vi "Begin.vi"   [LabVIEW 2012]
doc: "Called before other user functions, this VI is expected to open initial I/O refnums, load in file data, and do all program initialization. Notice that the <B>error out</B> terminal is simply used for data flow. Wiring it to other structures or subVIs ensures that this VI runs first."
uses:
  <vilib>/Rock Robotics/SystemInterfaces/Typedef/FPGA_TypedefAnalogModule.ctl
  <vilib>/Rock Robotics/SystemInterfaces/AI/FPGA_AIChannel.ctl
  <vilib>/Rock Robotics/SystemInterfaces/DIO/FPGA_DIOPWMChannel.ctl
  <vilib>/Rock Robotics/SystemInterfaces/Typedef/FPGA_TypedefDigitalModule.ctl
  <vilib>/Rock Robotics/SystemInterfaces/DIO/FPGA_DIOChannel.ctl
  <vilib>/Rock Robotics/WPI/Joystick/WPI_JoystickDeviceEnum.ctl
  <vilib>/Rock Robotics/SystemInterfaces/DIO/FPGA_DIORelayChannel.ctl
  <vilib>/Rock Robotics/WPI/Relay/WPI_RelayDirection.ctl
  <vilib>/Rock Robotics/WPI/SafetyOutput/WPI_SafetyOutputConfigMenu.ctl
  <vilib>/Rock Robotics/WPI/MotorControl/WPI_MotorControlOpen Jaguar.vi
  <vilib>/Rock Robotics/WPI/MotorControl/WPI_MotorControlOpen Victor.vi
  <vilib>/Rock Robotics/WPI/RobotDrive/WPI_RobotDriveOpen2MotorWithJaguar.vi
types:
  T1 = typedef "WPI_SafetyOutputConfigMenu.ctl" = enum16{"Enable", "Disable"}
  T2 = typedef "FPGA_DIOPWMChannel.ctl" = enum8{"PWM 1", "PWM 2", "PWM 3", "PWM 4", "PWM 5", "PWM 6", "PWM 7", "PWM 8", "PWM 9", "PWM 10", "Invalid"}
  T3 = typedef "WPI_RobotDriveDevRef.ctl" = cluster{"DevStatus":errorcluster, "Motors[]":T4[], "Square Inputs":bool, "Max Output":dbl, "Isochronous":bool}
  T4 = typedef "WPI_MotorControlDeviceRef.ctl" = cluster{"DeviceStatus":errorcluster, "Type":enum16{"PWM", "CAN"}, "PWM":cluster{"Digital Module":T5, "PWM Channel":T2, "DeadBand":T6}, "CAN":cluster{"Device Number":u8, "Control Mode":T7, "Semaphore":T8, "Max Vout":dbl}, "Invert":bool, "TransformRef":T9, "InvTransformRef":T9}
  T5 = typedef "FPGA_TypedefDigitalModule.ctl" = enum16{"Digital Module 1", "Digital Module 2"}
  T6 = typedef "WPI_PWMDeadband.ctl" = cluster{"Name":string, "maxPositivePwm":i32, "minPositivePwm":i32, "centerPwm":i32, "maxNegativePwm":i32, "minNegativePwm":i32, "angularRange":u16}
  T7 = typedef "WPI_CANJaguar_ControlMode.ctl" = enum8{"Percent VBus", "Current", "Speed", "Position", "Voltage"}
  T8 = typedef "Semaphore RefNum" = refnum<k1>
  T9 = typedef "WPI_PWMTransform_ConPane.ctl" = refnum<vi>
  T10 = typedef "WPI_RelayDirection.ctl" = enum16{"Both directions", "Forward only", "Reverse only"}
  T11 = typedef "FPGA_DIORelayChannel.ctl" = enum8{"Relay 1", "Relay 2", "Relay 3", "Relay 4", "Relay 5", "Relay 6", "Relay 7", "Relay 8", "Invalid"}
  T12 = typedef "WPI_ServoDeviceRef.ctl" = cluster{"DeviceStatus":errorcluster, "Digital Module":T5, "PWM Channel":T2, "DeadBand":T6}
  T13 = typedef "WPI_RelayDevRef.ctl" = cluster{"DevStatus":errorcluster, "Relay Channel":T11, "Digital Module":T5, "Relay Direction":T10}
  T14 = typedef "WPI_JoystickDeviceEnum.ctl" = enum16{"USB 1", "USB 2", "USB 3", "USB 4", "Kinect 1", "Kinect 2"}
  T15 = typedef "WPI_JoystickDevRef.ctl" = cluster{"Device":T14}
  T16 = typedef "FPGA_DIOChannel.ctl" = enum8{"DIO 1", "DIO 2", "DIO 3", "DIO 4", "DIO 5", "DIO 6", "DIO 7", "DIO 8", "DIO 9", "DIO 10", "DIO 11", "DIO 12", "DIO 13", "DIO 14", "Invalid"}
  T17 = typedef "WPI_DigitalInputDevRef.ctl" = cluster{"DevStatus":errorcluster, "DIO Channel":T16, "Digital Module":T5}
  T18 = typedef "FPGA_AIChannel.ctl" = enum8{"AI 1", "AI 2", "AI 3", "AI 4", "AI 5", "AI 6", "AI 7", "AI 8", "Invalid"}
  T19 = typedef "FPGA_TypedefAnalogModule.ctl" = enum16{"Analog Module 1", "Analog Module 2"}
  T20 = typedef "WPI_AnalogChannelDevRef.ctl" = cluster{"DevStatus":errorcluster, "Analog Module":T19, "Analog Channel":T18}
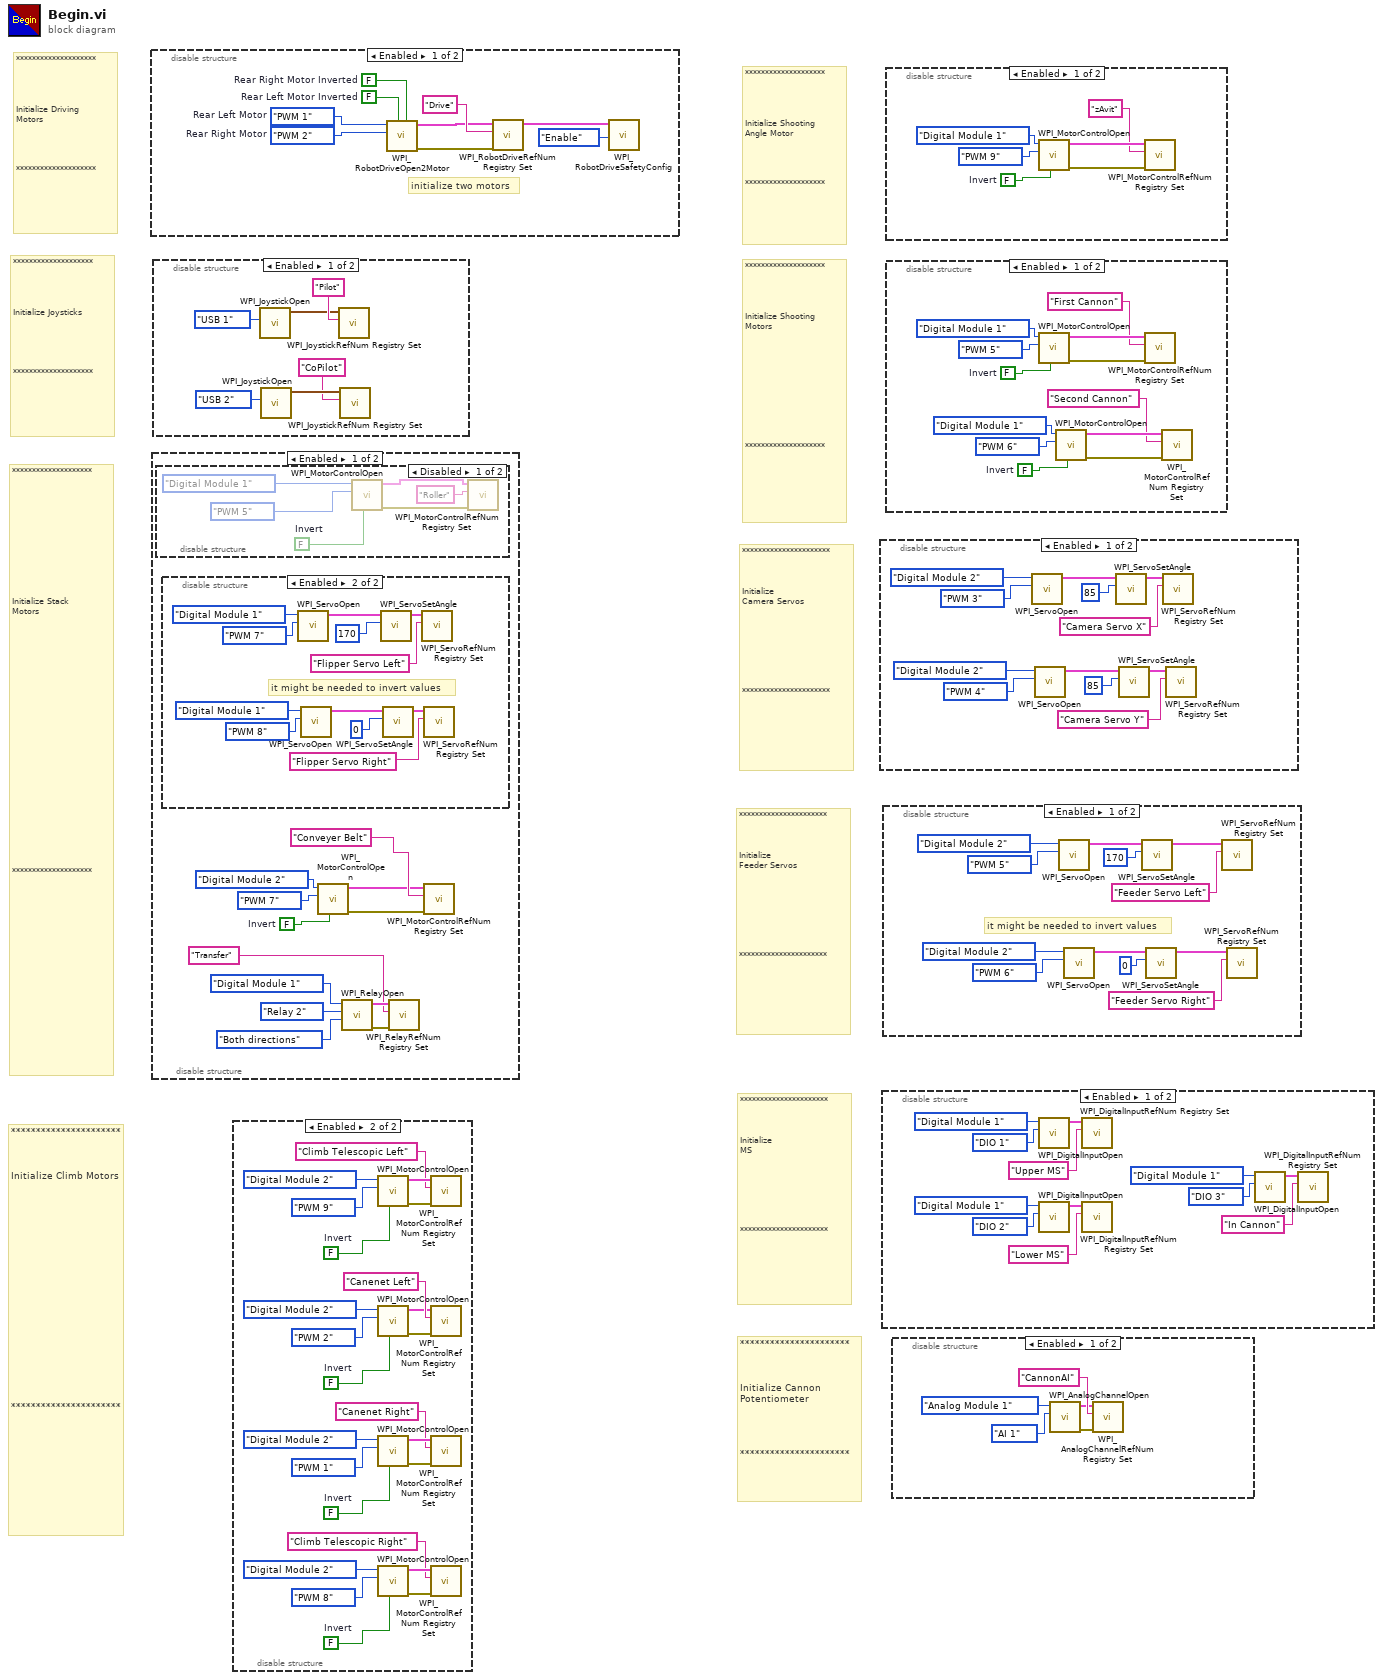
[diagram p0: block diagram]
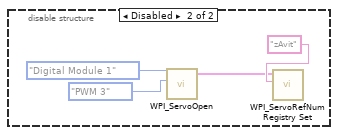
[diagram p7: hidden frame]
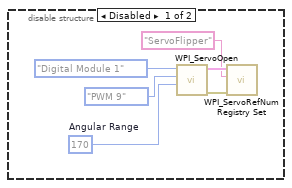
[diagram p11: hidden frame]
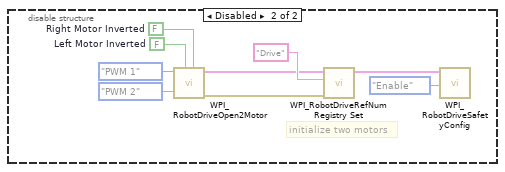
[diagram p13: hidden frame]
diagram:
  # "**********************\n\n\n           \nInitialize Cannon Potentiometer\n\n\n\n\n**********************"
  # "**********************\n\n\n\nInitialize\nMS\n\n\n\n\n\n\n\n**********************"
  # "**********************\n\n\n\nInitialize\nFeeder Servos\n\n\n\n\n\n\n\n\n**********************"
  # "**********************\n\n\n\nInitialize\nCamera Servos\n\n\n\n\n\n\n\n\n**********************"
  # "**********************\n\n\n\nInitialize Climb Motors          \n\n\n\n\n\n\n\n\n\n\n\n\n\n\n\n\n\n\n\n\n**********************"
  # "********************\n\n\n\n\nInitialize Shooting\nAngle Motor\n\n\n\n\n********************"
  # "********************\n\n\n\n\nInitialize Shooting\nMotors\n\n\n\n\n\n\n\n\n\n\n\n********************"
  # "********************\n\n\n\n\n\n\n\n\n\n\n\n\nInitialize Stack \nMotors\n\n\n\n\n\n\n\n\n\n\n\n\n\n\n\n\n\n\n\n\n\n\n\n\n\n********************"
  # "********************\n\n\n\n\nInitialize Driving\nMotors\n\n\n\n\n********************"
  # "********************\n\n\n\n\nInitialize Joysticks\n\n\n\n\n\n********************"
  n1 = disable-structure shown="Enabled" {
    frame Enabled {
      w1 = FPGA_DIOPWMChannel."PWM 2"  # Rear Right Motor
      w2 = FPGA_DIOPWMChannel."PWM 1"  # Rear Left Motor
      w3 = FALSE  # Rear Right Motor Inverted
      w4 = FALSE  # Rear Left Motor Inverted
      # "initialize two motors"
      n2 = call-poly <vilib>:"WPI_RobotDriveOpen2Motor.vi"("Right Motor Inverted"=w3, "Left Motor Inverted"=w4, "Right Motor"=w1, "Left Motor"=w2) -> ("error out"=w5:errorcluster, "RobotDriveDevRef"=w6:T3)  [unwired: 6 in]
      n3 = call <vilib>:"WPI_RobotDriveRefNum Registry Set.vi"("error in (no error)"=w5, "refnum name"="Drive", "RobotDriveDevRef"=w6) -> ("RobotDriveDevRef"=w8:T3)  [unwired: 8 out]
      n4 = call <vilib>:"WPI_RobotDriveSafetyConfig.vi"("mode"=WPI_SafetyOutputConfigMenu."Enable", "RobotDriveDevRef"=w8) -> ()  [unwired: 8 in, 2 out]
    }
    frame Disabled {
      w10 = FALSE  # Right Motor Inverted
      w11 = FALSE  # Left Motor Inverted
      # "initialize two motors"
      n5 = call-poly <vilib>:"WPI_RobotDriveOpen2Motor.vi"("Right Motor Inverted"=w10, "Left Motor Inverted"=w11, "Right Motor"=FPGA_DIOPWMChannel."PWM 2", "Left Motor"=FPGA_DIOPWMChannel."PWM 1") -> ("error out"=w14:errorcluster, "RobotDriveDevRef"=w15:T3)  [unwired: 6 in]
      n6 = call <vilib>:"WPI_RobotDriveRefNum Registry Set.vi"("error in (no error)"=w14, "refnum name"="Drive", "RobotDriveDevRef"=w15) -> ("RobotDriveDevRef"=w17:T3)  [unwired: 8 out]
      n7 = call <vilib>:"WPI_RobotDriveSafetyConfig.vi"("mode"=WPI_SafetyOutputConfigMenu."Enable", "RobotDriveDevRef"=w17) -> ()  [unwired: 8 in, 2 out]
    }
  }
  n8 = disable-structure shown="Enabled" {
    frame Enabled {
      w20 = FALSE  # Invert
      n9 = disable-structure shown="Disabled" {
        frame Disabled {
          w32 = FALSE  # Invert
          n10 = call-poly <vilib>:"WPI_MotorControlOpen.vi"("Invert"=w32, "PWM Channel"=FPGA_DIOPWMChannel."PWM 5", "Digital Module (Module 1)"=FPGA_TypedefDigitalModule."Digital Module 1") -> ("error out"=w31:errorcluster, "MotorControlDeviceRef"=w36:T4)  [unwired: 7 in]
          n11 = call <vilib>:"WPI_MotorControlRefNum Registry Set.vi"("error in (no error)"=w31, "refnum name"="Roller", "MotorControlDevRef"=w36) -> ()  [unwired: 7 in, 2 out]
        }
        frame Enabled {
        }
      }
      n12 = disable-structure shown="Enabled" {
        frame Disabled {
          w39 = u16 170  # Angular Range
          n13 = call <vilib>:"WPI_ServoOpen.vi"("Angular Range"=w39, "PWM Channel"=FPGA_DIOPWMChannel."PWM 9", "Digital Module (Module 1)"=FPGA_TypedefDigitalModule."Digital Module 1") -> ("error out"=w38:errorcluster, "ServoDeviceRef"=w42:T12)  [unwired: 7 in]
          n14 = call <vilib>:"WPI_ServoRefNum Registry Set.vi"("error in (no error)"=w38, "refnum name"="ServoFlipper", "ServoDeviceRef"=w42) -> ()  [unwired: 7 in, 2 out]
        }
        frame Enabled {
          # "it might be needed to invert values"
          n15 = call <vilib>:"WPI_ServoOpen.vi"("PWM Channel"=FPGA_DIOPWMChannel."PWM 7", "Digital Module (Module 1)"=FPGA_TypedefDigitalModule."Digital Module 1") -> ("ServoDeviceRef"=w54:T12)  [unwired: 8 in, 1 out]
          n16 = call <vilib>:"WPI_ServoOpen.vi"("PWM Channel"=FPGA_DIOPWMChannel."PWM 8", "Digital Module (Module 1)"=FPGA_TypedefDigitalModule."Digital Module 1") -> ("ServoDeviceRef"=w44:T12)  [unwired: 8 in, 1 out]
          n17 = call <vilib>:"WPI_ServoSetAngle.vi"("Angle"=170, "ServoDeviceRef"=w54) -> ("ServoDeviceRef"=w50:T12)  [unwired: 8 in, 1 out]
          n18 = call <vilib>:"WPI_ServoSetAngle.vi"("Angle"=0, "ServoDeviceRef"=w44) -> ("ServoDeviceRef"=w47:T12)  [unwired: 8 in, 1 out]
          n19 = call <vilib>:"WPI_ServoRefNum Registry Set.vi"("refnum name"="Flipper Servo Left", "ServoDeviceRef"=w50) -> ()  [unwired: 8 in, 2 out]
          n20 = call <vilib>:"WPI_ServoRefNum Registry Set.vi"("refnum name"="Flipper Servo Right", "ServoDeviceRef"=w47) -> ()  [unwired: 8 in, 2 out]
        }
      }
      n21 = call-poly <vilib>:"WPI_MotorControlOpen.vi"("Invert"=w20, "PWM Channel"=FPGA_DIOPWMChannel."PWM 7", "Digital Module (Module 1)"=FPGA_TypedefDigitalModule."Digital Module 2") -> ("error out"=w19:errorcluster, "MotorControlDeviceRef"=w23:T4)  [unwired: 7 in]
      n22 = call <vilib>:"WPI_RelayOpen.vi"("Relay Direction"=WPI_RelayDirection."Both directions", "Relay Channel"=FPGA_DIORelayChannel."Relay 2", "Digital Module (Module 1)"=FPGA_TypedefDigitalModule."Digital Module 1") -> ("error out"=w27:errorcluster, "RelayDevRef"=w26:T13)  [unwired: 7 in]
      n23 = call <vilib>:"WPI_RelayRefNum Registry Set.vi"("error in (no error)"=w27, "refnum name"="Transfer", "RelayDevRef"=w26) -> ()  [unwired: 7 in, 2 out]
      n24 = call <vilib>:"WPI_MotorControlRefNum Registry Set.vi"("error in (no error)"=w19, "refnum name"="Conveyer Belt", "MotorControlDevRef"=w23) -> ()  [unwired: 7 in, 2 out]
    }
    frame Disabled {
    }
  }
  n25 = disable-structure shown="Enabled" {
    frame Enabled {
      n26 = call <vilib>:"WPI_JoystickOpen.vi"("JoystickDevice"=WPI_JoystickDeviceEnum."USB 1") -> ("JoystickDevRef"=w59:T15)  [unwired: 10 in]
      n27 = call <vilib>:"WPI_JoystickOpen.vi"("JoystickDevice"=WPI_JoystickDeviceEnum."USB 2") -> ("JoystickDevRef"=w56:T15)  [unwired: 10 in]
      n28 = call <vilib>:"WPI_JoystickRefNum Registry Set.vi"("refnum name"="Pilot", "JoystickDevRef"=w59) -> ()  [unwired: 8 in, 2 out]
      n29 = call <vilib>:"WPI_JoystickRefNum Registry Set.vi"("refnum name"="CoPilot", "JoystickDevRef"=w56) -> ()  [unwired: 8 in, 2 out]
    }
    frame Disabled {
    }
  }
  n30 = disable-structure shown="Enabled" {
    frame Disabled {
    }
    frame Enabled {
      w64 = FALSE  # Invert
      w71 = FALSE  # Invert
      w77 = FALSE  # Invert
      w80 = FALSE  # Invert
      n31 = call-poly <vilib>:"WPI_MotorControlOpen.vi"("Invert"=w64, "PWM Channel"=FPGA_DIOPWMChannel."PWM 9", "Digital Module (Module 1)"=FPGA_TypedefDigitalModule."Digital Module 2") -> ("error out"=w63:errorcluster, "MotorControlDeviceRef"=w67:T4)  [unwired: 7 in]
      n32 = call-poly <vilib>:"WPI_MotorControlOpen.vi"("Invert"=w77, "PWM Channel"=FPGA_DIOPWMChannel."PWM 2", "Digital Module (Module 1)"=FPGA_TypedefDigitalModule."Digital Module 2") -> ("error out"=w78:errorcluster, "MotorControlDeviceRef"=w73:T4)  [unwired: 7 in]
      n33 = call-poly <vilib>:"WPI_MotorControlOpen.vi"("Invert"=w80, "PWM Channel"=FPGA_DIOPWMChannel."PWM 1", "Digital Module (Module 1)"=FPGA_TypedefDigitalModule."Digital Module 2") -> ("error out"=w79:errorcluster, "MotorControlDeviceRef"=w84:T4)  [unwired: 7 in]
      n34 = call-poly <vilib>:"WPI_MotorControlOpen.vi"("Invert"=w71, "PWM Channel"=FPGA_DIOPWMChannel."PWM 8", "Digital Module (Module 1)"=FPGA_TypedefDigitalModule."Digital Module 2") -> ("error out"=w72:errorcluster, "MotorControlDeviceRef"=w68:T4)  [unwired: 7 in]
      n35 = call <vilib>:"WPI_MotorControlRefNum Registry Set.vi"("error in (no error)"=w63, "refnum name"="Climb Telescopic Left", "MotorControlDevRef"=w67) -> ()  [unwired: 7 in, 2 out]
      n36 = call <vilib>:"WPI_MotorControlRefNum Registry Set.vi"("error in (no error)"=w78, "refnum name"="Canenet Left", "MotorControlDevRef"=w73) -> ()  [unwired: 7 in, 2 out]
      n37 = call <vilib>:"WPI_MotorControlRefNum Registry Set.vi"("error in (no error)"=w79, "refnum name"="Canenet Right", "MotorControlDevRef"=w84) -> ()  [unwired: 7 in, 2 out]
      n38 = call <vilib>:"WPI_MotorControlRefNum Registry Set.vi"("error in (no error)"=w72, "refnum name"="Climb Telescopic Right", "MotorControlDevRef"=w68) -> ()  [unwired: 7 in, 2 out]
    }
  }
  n39 = disable-structure shown="Enabled" {
    frame Enabled {
      n40 = call <vilib>:"WPI_ServoOpen.vi"("PWM Channel"=FPGA_DIOPWMChannel."PWM 3", "Digital Module (Module 1)"=FPGA_TypedefDigitalModule."Digital Module 2") -> ("ServoDeviceRef"=w93:T12)  [unwired: 8 in, 1 out]
      n41 = call <vilib>:"WPI_ServoOpen.vi"("PWM Channel"=FPGA_DIOPWMChannel."PWM 4", "Digital Module (Module 1)"=FPGA_TypedefDigitalModule."Digital Module 2") -> ("ServoDeviceRef"=w88:T12)  [unwired: 8 in, 1 out]
      n42 = call <vilib>:"WPI_ServoSetAngle.vi"("Angle"=85, "ServoDeviceRef"=w93) -> ("ServoDeviceRef"=w92:T12)  [unwired: 8 in, 1 out]
      n43 = call <vilib>:"WPI_ServoSetAngle.vi"("Angle"=85, "ServoDeviceRef"=w88) -> ("ServoDeviceRef"=w89:T12)  [unwired: 8 in, 1 out]
      n44 = call <vilib>:"WPI_ServoRefNum Registry Set.vi"("refnum name"="Camera Servo X", "ServoDeviceRef"=w92) -> ()  [unwired: 8 in, 2 out]
      n45 = call <vilib>:"WPI_ServoRefNum Registry Set.vi"("refnum name"="Camera Servo Y", "ServoDeviceRef"=w89) -> ()  [unwired: 8 in, 2 out]
    }
    frame Disabled {
    }
  }
  n46 = disable-structure shown="Enabled" {
    frame Enabled {
      n47 = call <vilib>:"WPI_DigitalInputOpen.vi"("DIO Channel"=FPGA_DIOChannel."DIO 1", "Digital Module (Module 1)"=FPGA_TypedefDigitalModule."Digital Module 1") -> ("DigitalInputDevRef"=w101:T17)  [unwired: 8 in, 1 out]
      n48 = call <vilib>:"WPI_DigitalInputOpen.vi"("DIO Channel"=FPGA_DIOChannel."DIO 2", "Digital Module (Module 1)"=FPGA_TypedefDigitalModule."Digital Module 1") -> ("DigitalInputDevRef"=w108:T17)  [unwired: 8 in, 1 out]
      n49 = call <vilib>:"WPI_DigitalInputRefNum Registry Set.vi"("refnum name"="Upper MS", "DigitalInputDevRef"=w101) -> ()  [unwired: 8 in, 2 out]
      n50 = call <vilib>:"WPI_DigitalInputRefNum Registry Set.vi"("refnum name"="Lower MS", "DigitalInputDevRef"=w108) -> ()  [unwired: 8 in, 2 out]
      n51 = call <vilib>:"WPI_DigitalInputOpen.vi"("DIO Channel"=FPGA_DIOChannel."DIO 3", "Digital Module (Module 1)"=FPGA_TypedefDigitalModule."Digital Module 1") -> ("DigitalInputDevRef"=w97:T17)  [unwired: 8 in, 1 out]
      n52 = call <vilib>:"WPI_DigitalInputRefNum Registry Set.vi"("refnum name"="In Cannon", "DigitalInputDevRef"=w97) -> ()  [unwired: 8 in, 2 out]
    }
    frame Disabled {
    }
  }
  n53 = disable-structure shown="Enabled" {
    frame Enabled {
      # "it might be needed to invert values"
      n54 = call <vilib>:"WPI_ServoOpen.vi"("PWM Channel"=FPGA_DIOPWMChannel."PWM 5", "Digital Module (Module 1)"=FPGA_TypedefDigitalModule."Digital Module 2") -> ("ServoDeviceRef"=w117:T12)  [unwired: 8 in, 1 out]
      n55 = call <vilib>:"WPI_ServoOpen.vi"("PWM Channel"=FPGA_DIOPWMChannel."PWM 6", "Digital Module (Module 1)"=FPGA_TypedefDigitalModule."Digital Module 2") -> ("ServoDeviceRef"=w116:T12)  [unwired: 8 in, 1 out]
      n56 = call <vilib>:"WPI_ServoSetAngle.vi"("Angle"=170, "ServoDeviceRef"=w117) -> ("ServoDeviceRef"=w112:T12)  [unwired: 8 in, 1 out]
      n57 = call <vilib>:"WPI_ServoSetAngle.vi"("Angle"=0, "ServoDeviceRef"=w116) -> ("ServoDeviceRef"=w111:T12)  [unwired: 8 in, 1 out]
      n58 = call <vilib>:"WPI_ServoRefNum Registry Set.vi"("refnum name"="Feeder Servo Left", "ServoDeviceRef"=w112) -> ()  [unwired: 8 in, 2 out]
      n59 = call <vilib>:"WPI_ServoRefNum Registry Set.vi"("refnum name"="Feeder Servo Right", "ServoDeviceRef"=w111) -> ()  [unwired: 8 in, 2 out]
    }
    frame Disabled {
    }
  }
  n60 = disable-structure shown="Enabled" {
    frame Enabled {
      w122 = FALSE  # Invert
      n61 = call-poly <vilib>:"WPI_MotorControlOpen.vi"("Invert"=w122, "PWM Channel"=FPGA_DIOPWMChannel."PWM 9", "Digital Module (Module 1)"=FPGA_TypedefDigitalModule."Digital Module 1") -> ("error out"=w121:errorcluster, "MotorControlDeviceRef"=w126:T4)  [unwired: 7 in]
      n62 = call <vilib>:"WPI_MotorControlRefNum Registry Set.vi"("error in (no error)"=w121, "refnum name"="zAvit", "MotorControlDevRef"=w126) -> ()  [unwired: 7 in, 2 out]
    }
    frame Disabled {
      n63 = call <vilib>:"WPI_ServoOpen.vi"("PWM Channel"=FPGA_DIOPWMChannel."PWM 3", "Digital Module (Module 1)"=FPGA_TypedefDigitalModule."Digital Module 1") -> ("ServoDeviceRef"=w127:T12)  [unwired: 8 in, 1 out]
      n64 = call <vilib>:"WPI_ServoRefNum Registry Set.vi"("refnum name"="zAvit", "ServoDeviceRef"=w127) -> ()  [unwired: 8 in, 2 out]
    }
  }
  n65 = disable-structure shown="Enabled" {
    frame Enabled {
      w132 = FALSE  # Invert
      w138 = FALSE  # Invert
      n66 = call-poly <vilib>:"WPI_MotorControlOpen.vi"("Invert"=w138, "PWM Channel"=FPGA_DIOPWMChannel."PWM 5", "Digital Module (Module 1)"=FPGA_TypedefDigitalModule."Digital Module 1") -> ("error out"=w137:errorcluster, "MotorControlDeviceRef"=w142:T4)  [unwired: 7 in]
      n67 = call-poly <vilib>:"WPI_MotorControlOpen.vi"("Invert"=w132, "PWM Channel"=FPGA_DIOPWMChannel."PWM 6", "Digital Module (Module 1)"=FPGA_TypedefDigitalModule."Digital Module 1") -> ("error out"=w131:errorcluster, "MotorControlDeviceRef"=w136:T4)  [unwired: 7 in]
      n68 = call <vilib>:"WPI_MotorControlRefNum Registry Set.vi"("error in (no error)"=w137, "refnum name"="First Cannon", "MotorControlDevRef"=w142) -> ()  [unwired: 7 in, 2 out]
      n69 = call <vilib>:"WPI_MotorControlRefNum Registry Set.vi"("error in (no error)"=w131, "refnum name"="Second Cannon", "MotorControlDevRef"=w136) -> ()  [unwired: 7 in, 2 out]
    }
    frame Disabled {
    }
  }
  n70 = disable-structure shown="Enabled" {
    frame Enabled {
      n71 = call <vilib>:"WPI_AnalogChannelOpen.vi"("Analog Channel"=FPGA_AIChannel."AI 1", "Analog Module (Module 1)"=FPGA_TypedefAnalogModule."Analog Module 1") -> ("error out"=w144:errorcluster, "AIDeviceRef"=w143:T20)  [unwired: 8 in]
      n72 = call <vilib>:"WPI_AnalogChannelRefNum Registry Set.vi"("error in (no error)"=w144, "refnum name"="CannonAI", "AIDeviceRef"=w143) -> ()  [unwired: 7 in, 2 out]
    }
    frame Disabled {
    }
  }
